vi "Scaling Coefficients from INI.vi"(8 "error in":errorcluster, 11 "Config Refnum in":T2) -> (0 "error out":errorcluster, 3 "Config Refnum out":T2, 4 "Scaling Coefficients":T1)   [LabVIEW 2018, in "AE75TX Actor.lvlib" / "AE75TX.lvclass"]
uses:
  AE75TX.lvclass
  <vilib>/Utility/config.llb/Config Data RefNum.ctl
  Controls/Scaling Coefficients Measurements.ctl
  <vilib>/Utility/config.llb/Read Key (Double).vi
  <vilib>/Utility/config.llb/NI_LVConfig.lvlib
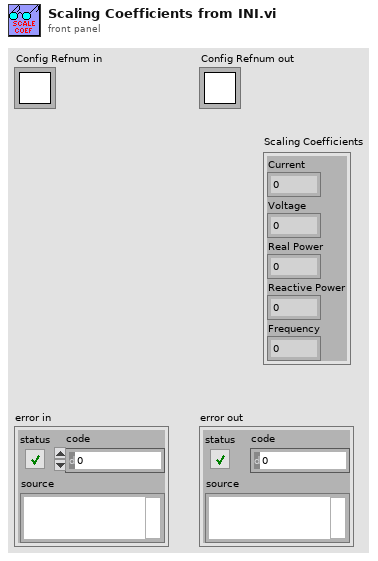
[diagram p1: front panel]
types:
  T1 = typedef "AE75TX Actor.lvlib/AE75TX.lvclass/Scaling Coefficients Measurements.ctl" = cluster{"Current":dbl, "Voltage":dbl, "Real Power":dbl, "Reactive Power":dbl, "Frequency":dbl}
  T2 = typedef "NI_LVConfig.lvlib/Config Data RefNum.ctl" = refnum<k1>
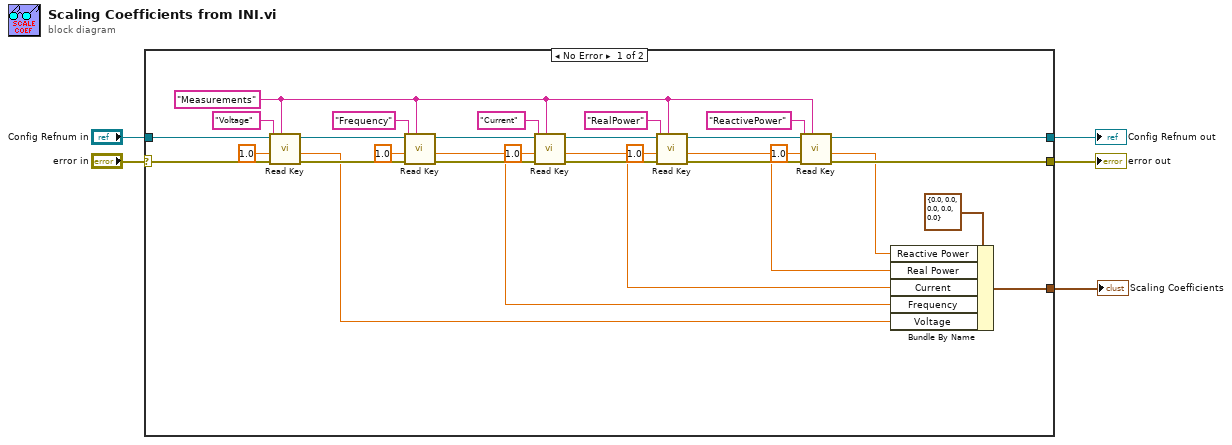
[diagram p0: block diagram]
diagram:
  n1 = case shown="No Error" "error in" {
    selector: "error in" -> [w32 w37]
    tunnel: [w35 _] -> w1
    tunnel: [w21 w37] -> w5
    tunnel: [w20 w36] -> w4
    tunnel: "Config Refnum in" -> [w31 w36]
    frame No Error {
      w12 = "Measurements" ("section")
      n2 = call-poly <vilib>:"Read Key.vi"("section"=w12, "error in (no error)"=w32, "default value"=1.0, "key"="Voltage", "refnum"=w31) -> ("error out"=w34:errorcluster, "value"=w6:dbl, "refnum out"=w33:T2)  [unwired: 3 in, 1 out]
      n3 = call-poly <vilib>:"Read Key.vi"("section"=w12, "error in (no error)"=w34, "default value"=1.0, "key"="Frequency", "refnum"=w33) -> ("error out"=w25:errorcluster, "value"=w7:dbl, "refnum out"=w24:T2)  [unwired: 3 in, 1 out]
      n4 = call-poly <vilib>:"Read Key.vi"("section"=w12, "error in (no error)"=w25, "default value"=1.0, "key"="Current", "refnum"=w24) -> ("error out"=w27:errorcluster, "value"=w8:dbl, "refnum out"=w26:T2)  [unwired: 3 in, 1 out]
      n5 = call-poly <vilib>:"Read Key.vi"("section"=w12, "error in (no error)"=w27, "default value"=1.0, "key"="RealPower", "refnum"=w26) -> ("error out"=w29:errorcluster, "value"=w9:dbl, "refnum out"=w28:T2)  [unwired: 3 in, 1 out]
      n6 = call-poly <vilib>:"Read Key.vi"("section"=w12, "error in (no error)"=w29, "default value"=1.0, "key"="ReactivePower", "refnum"=w28) -> ("error out"=w21:errorcluster, "value"=w10:dbl, "refnum out"=w20:T2)  [unwired: 3 in, 1 out]
      n7 = Bundle By Name(cluster=T1 {"Current"=0.0, "Voltage"=0.0, "Real Power"=0.0, "Reactive Power"=0.0, "Frequency"=0.0} ("Measurements"), "Reactive Power"=w10, "Real Power"=w9, "Current"=w8, "Frequency"=w7, "Voltage"=w6) -> (w35:T1)
    }
    frame Error {
    }
  }
  "error out" <- w5
  "Config Refnum out" <- w4
  "Scaling Coefficients" <- w1
